vi "openbci_read.vi"(8 "error in":errorcluster, 10 "N samples (2)":i32=2, 11 "OBCI dev in":T1={"COM port"="", "n_ch (8)"=enum."8 Channels", "delay_tx"=50}) -> (0 "error out":errorcluster, 1 "Acc data":dbl[][](array[numeric]), 2 "EEG data":dbl[][](array[numeric]), 3 "OBCI dev out":T1={"COM port"="", "n_ch (8)"=enum."8 Channels", "delay_tx"=50})   [LabVIEW 2013]
doc: "Read and parse data packages.\nIdentifies Header, Data and Footer. The output of this VI is an sample of EEG data (8 channels) and Accelerometer data if it's present in the package.\nIn case of 16 channels the array will be ordered by eeg_order_8ch_16ch.vi"
uses:
  Control Def/openbci_device.ctl
  Control Def/channel_count.ctl
  Control Def/package_parts.ctl
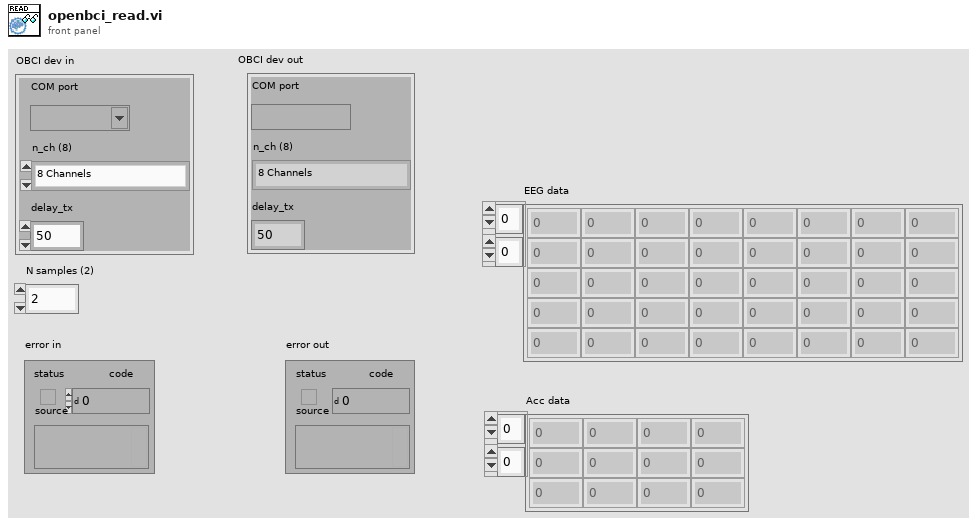
[diagram p1: front panel]
types:
  T1 = typedef "openbci_device.ctl" = cluster{"COM port":refnum<visa-resource-name>, "n_ch (8)":T2, "delay_tx":u32}
  T2 = typedef "channel_count.ctl" = enum16{"8 Channels", "16 Channels"}
  T3 = typedef "package_parts.ctl" = enum16{"Header", "EEG_data", "ACC_data", "Footer"}
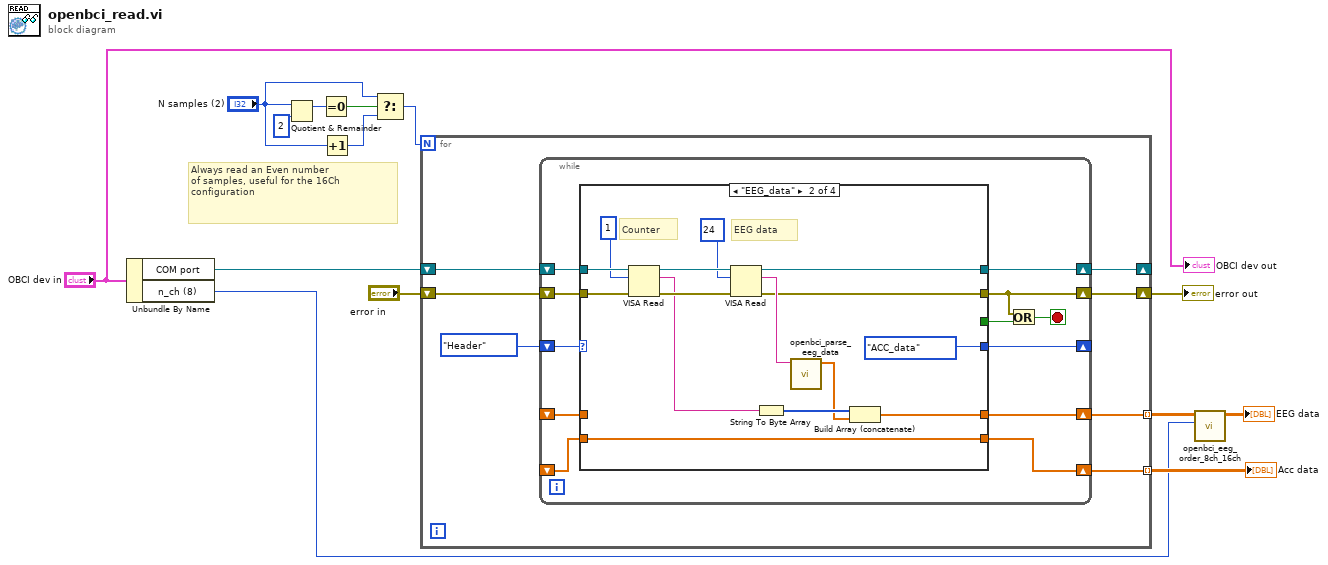
[diagram p0: block diagram]
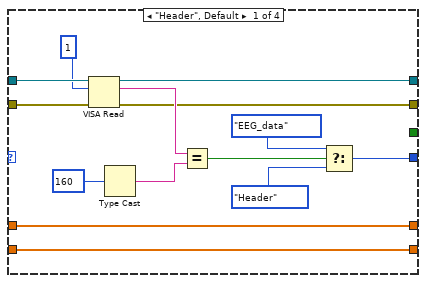
[diagram p2: hidden frame]
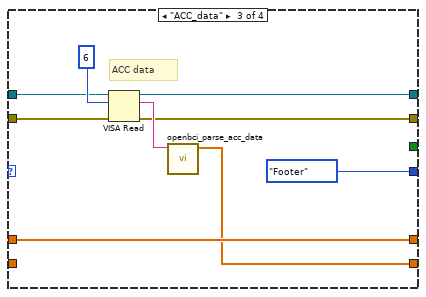
[diagram p3: hidden frame]
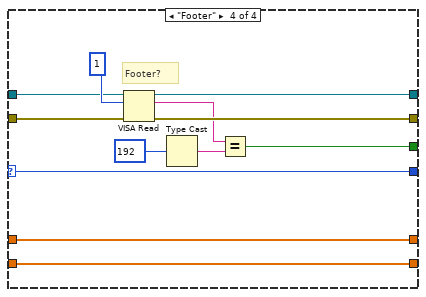
[diagram p4: hidden frame]
diagram:
  # "Always read an Even number\nof samples, useful for the 16Ch\nconfiguration"
  n1 = Unbundle By Name("OBCI dev in") -> ("COM port"=w11:refnum<visa-resource-name>, "n_ch (8)"=w2:T2)
  n2 = Quotient & Remainder(x="N samples (2)", y=2) -> (x-y*floor(x/y)=w9:i32)  [unwired: 1 out]
  n3 = Equal To 0?(x=w9) -> (x = 0?=w8:bool)
  n4 = Increment(x="N samples (2)") -> (x+1=w7:i32)
  n5 = Select(t="N samples (2)", s=w8, f=w7) -> (s? t:f=w5:i32)
  n6 = for {
    N: w5 -> [_]
    shift-right: [w19] -> _
    shift-left: w11 -> [w21]
    shift-right: [w17] -> w13
    shift-left: "error in" -> [w18]
    tunnel: [w16] -> w4 mode=indexing
    tunnel: [w15] -> w12 mode=indexing
    n7 = while {
      shift-right: [w30] -> _
      shift-left: package_parts."Header" -> [w33]
      shift-right: [w31] -> w19
      shift-left: w21 -> [w32]
      shift-right: [w23] -> w17
      shift-left: w18 -> [w29]
      shift-right: [w28] -> w16
      shift-left: _ -> [w27]
      shift-right: [w26] -> w15
      shift-left: _ -> [w25]
      stop <- w24 stop-if-true
      n8 = case shown="\"EEG_data\"" w33 {
        selector: w33 -> [_ _ _ w74]
        tunnel: w32 -> [w47 w62 w69 w80]
        tunnel: [w45 w50 w64 w79] -> w31
        tunnel: [w39 package_parts."ACC_data" package_parts."Footer" w74] -> w30
        tunnel: w29 -> [w37 w57 w70 w77]
        tunnel: [w35 w49 w63 w78] -> w23
        tunnel: [w36 w52 w67 w83] -> w28
        tunnel: w27 -> [w36 _ w67 w83]
        tunnel: [w34 w51 w65 w82] -> w26
        tunnel: w25 -> [w34 w51 _ w82]
        tunnel: [_ _ _ w72] -> w22
        frame "Header", Default {
          n9 = VISA Read(VISA resource name=w47, byte count=u32 1, error in (no error)=w37) -> (VISA resource name out=w45:refnum<visa-resource-name>, read buffer=w44:string, error out=w35:errorcluster)  [unwired: 1 out]
          n10 = Type Cast(x=u8 160) -> (*(type *) &x=w42:string)  [unwired: 1 in]
          n11 = Equal?(x=w44, y=w42) -> (x = y?=w41:bool)
          n12 = Select(t=package_parts."EEG_data", s=w41, f=package_parts."Header") -> (s? t:f=w39:T3)
        }
        frame "EEG_data" {
          # "EEG data"
          # "Counter"
          n13 = VISA Read(VISA resource name=w62, byte count=u32 1, error in (no error)=w57) -> (VISA resource name out=w59:refnum<visa-resource-name>, read buffer=w56:string, error out=w60:errorcluster)  [unwired: 1 out]
          n14 = VISA Read(VISA resource name=w59, byte count=u32 24, error in (no error)=w60) -> (VISA resource name out=w50:refnum<visa-resource-name>, read buffer=w55:string, error out=w49:errorcluster)  [unwired: 1 out]
          n15 = String To Byte Array(string=w56) -> (unsigned byte array=w54:u8[])
          n16 = call "openbci_parse_eeg_data.vi"("string_eeg_data"=w55) -> ("eeg_data"=w53:dbl[])  [unwired: 10 in]
          n17 = Build Array (concatenate)(w54, w53) -> (w52:dbl[])
        }
        frame "ACC_data" {
          # "ACC data"
          n18 = VISA Read(VISA resource name=w69, byte count=u32 6, error in (no error)=w70) -> (VISA resource name out=w64:refnum<visa-resource-name>, read buffer=w66:string, error out=w63:errorcluster)  [unwired: 1 out]
          n19 = call "openbci_parse_acc_data.vi"("string_acc_data"=w66) -> ("acc_data"=w65:dbl[])  [unwired: 10 in]
        }
        frame "Footer" {
          # "Footer?"
          n20 = VISA Read(VISA resource name=w80, byte count=u32 1, error in (no error)=w77) -> (VISA resource name out=w79:refnum<visa-resource-name>, read buffer=w75:string, error out=w78:errorcluster)  [unwired: 1 out]
          n21 = Type Cast(x=u8 192) -> (*(type *) &x=w73:string)  [unwired: 1 in]
          n22 = Equal?(x=w75, y=w73) -> (x = y?=w72:bool)
        }
      }
      n23 = Or(x=w23, y=w22) -> (x .or. y?=w24:bool)
    }
  }
  "error out" <- w13
  "Acc data" <- w12
  n24 = call "openbci_eeg_order_8ch_16ch.vi"("n_ch (8)"=w2, "EEG data in"=w4) -> ("EEG data out"=→"EEG data":dbl[][])  [unwired: 9 in]
  "OBCI dev out" <- "OBCI dev in"
